vi "Shmove Shot Adjust.vi"(10 "Input Velocities":T1, 11 "Hub Distance":dbl) -> (3 "Adjusted Hub Distance":dbl)   [LabVIEW 2025]
uses:
  swerve-template/Type Definitions/Data/Robot Velocities.ctl
  Get Distance LUT.vi
panel:
  in  "TOF LUT (s)":dbl[](array[numeric])
  in  "Latency Compensation (s)":dbl=0.1
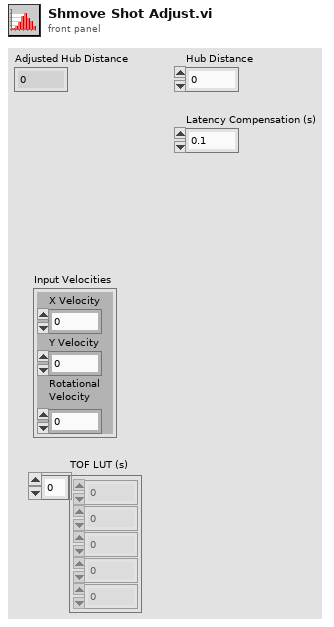
[diagram p1: front panel]
types:
  T1 = typedef "Robot Velocities.ctl" = cluster{"X Velocity":dbl, "Y Velocity":dbl, "Rotational \nVelocity":dbl}
  T2 = cluster{"Start Distance":i32, "Step Size":i32, "Max Distance":i32}
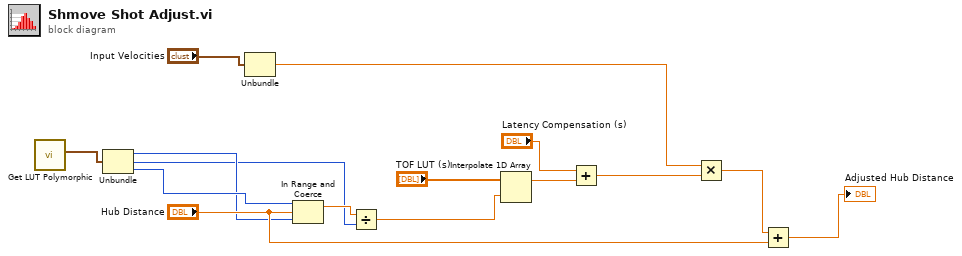
[diagram p0: block diagram]
diagram:
  n1 = call-poly "Get LUT Polymorphic.vi"() -> ("Info"=w5:T2)  [unwired: 10 in, 1 out]
  n2 = Unbundle(w5) -> ("Start Distance"=w2:i32, "Step Size"=w1:i32, "Max Distance"=w3:i32)
  n3 = Unbundle("Input Velocities") -> ("Y Velocity"=w9:dbl)  [unwired: 2 out]
  n4 = In Range and Coerce(upper limit=w3, x="Hub Distance", lower limit=w2) -> (coerced(x)=w14:dbl)  [unwired: 1 out]
  n5 = Divide(x=w14, y=w1) -> (x/y=w13:dbl)
  n6 = Interpolate 1D Array(1:w13, 2:"TOF LUT (s)") -> (0:w12:dbl)
  n7 = Add(x="Latency Compensation (s)", y=w12) -> (x+y=w8:dbl)
  n8 = Multiply(x=w9, y=w8) -> (x*y=w7:dbl)
  n9 = Add(x=w7, y="Hub Distance") -> (x+y=→"Adjusted Hub Distance":dbl)
